vi "ConfigureTrig.vi"(8 "error in (no error)":errorcluster, 11 "reference in":refnum<class "mmWave instrument.lvclass">) -> (0 "error out":errorcluster, 3 "reference out":refnum<class "mmWave instrument.lvclass">)   [LabVIEW 2019, in "mmWave instrument.lvclass"]
doc: "Configures triggering for device"
uses:
  mmWave instrument.lvclass
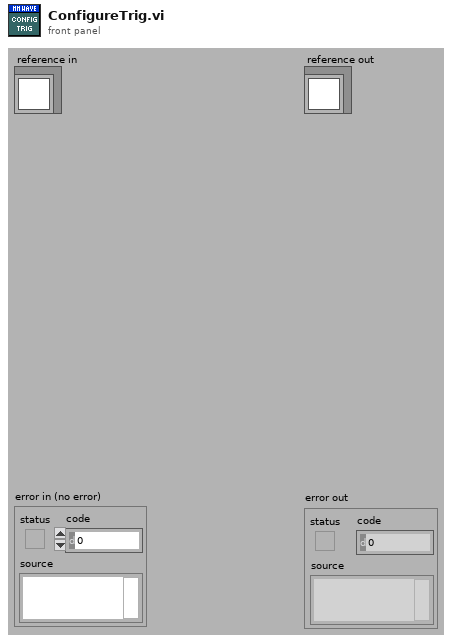
[diagram p1: front panel]
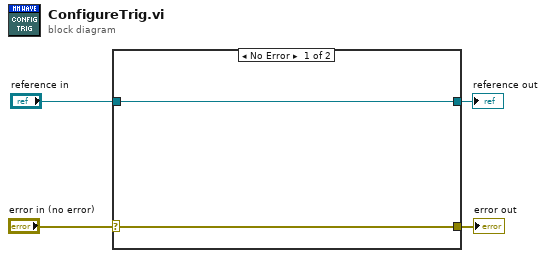
[diagram p0: block diagram]
diagram:
  n1 = case shown="No Error" "error in (no error)" {
    selector: "error in (no error)" -> [w6 w8]
    tunnel: [w6 w8] -> w3
    tunnel: [w5 w7] -> w1
    tunnel: "reference in" -> [w5 w7]
    frame No Error {
    }
    frame Error {
    }
  }
  "error out" <- w3
  "reference out" <- w1
